vi "Thingworx_Read.vi"(8 "error in (no error)":errorcluster, 10 "Property In":T3, 11 "Device in":T2) -> (0 "error out":errorcluster, 2 "Property":T3, 3 "Device Out":T2)   [LabVIEW 2016]
uses:
  _subVIs/Device.ctl
  _subVIs/HTTPComm.ctl
panel:
  out "Comm":T1
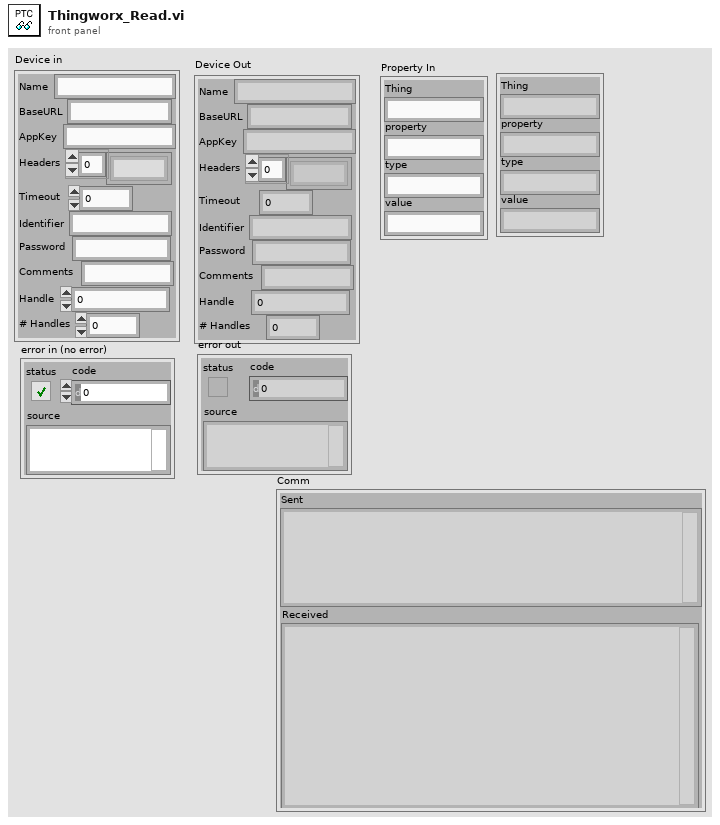
[diagram p1: front panel]
types:
  T1 = typedef "HTTPComm.ctl" = cluster{"url":string, "sent headers":string, "sent body":string, "headers":string, "body":string, "Sent":string, "Received":string}
  T2 = typedef "Device.ctl" = cluster{"Name":string, "BaseURL":string, "AppKey":string, "Headers":string[], "Timeout":i32, "Identifier":string, "Password":string, "Comments":string, "Handle":u32, "# Handles":i32}
  T3 = cluster{"Thing":string, "property":string, "type":string, "value":string}
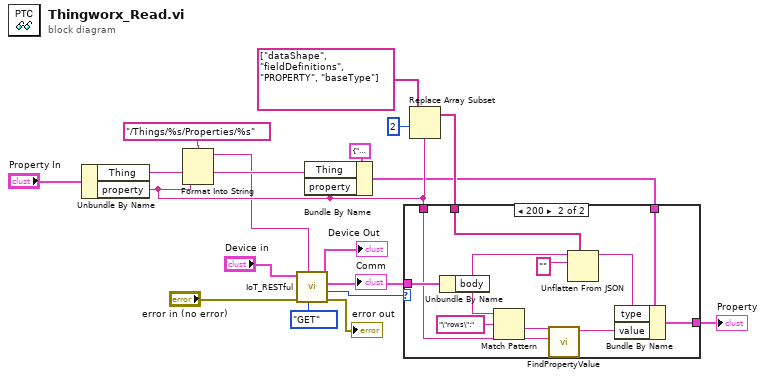
[diagram p0: block diagram]
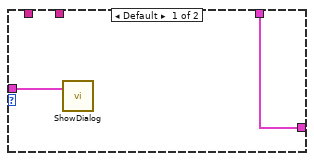
[diagram p2: hidden frame]
diagram:
  n1 = Unbundle By Name("Property In") -> ("Thing"=w11:string, "property"=w15:string)
  n2 = Format Into String(format string="/Things/%s/Properties/%s", w11, w15) -> (resulting string=w10:string)  [unwired: 2 in, 1 out]
  n3 = call "IoT_RESTful.vi"("Method"=enum16{"GET", "PUT", "POST", "MultiPOST"}."GET", "url"=w10, "error in"="error in (no error)", "Device In"="Device in") -> ("error out"=→"error out":errorcluster, "HTTP Code"=w17:i32, "Comm"=w7:T1, "Device Out"=→"Device Out":T2)  [unwired: 4 in]
  "Comm" <- w7
  n4 = Bundle By Name(cluster=T3 {"Thing"="", "property"="", "type"="", "value"=""} ("Property"), "Thing"=w11, "property"=w15) -> (w12:T3)
  n5 = Replace Array Subset(array=string[] ["dataShape", "fieldDefinitions", "PROPERTY", "baseType"] ("path"), new element=w15, index=2) -> (w16:string[])
  n6 = case shown="200" w17 {
    tunnel: w7 -> [w19 w31]
    tunnel: w12 -> [w20 w28]
    tunnel: [w20 w26] -> w2
    tunnel: w15 -> [_ w22]
    tunnel: w16 -> [_ w21]
    frame Default {
      n7 = call "ShowDialog.vi"("Comm"=w19) -> ()  [unwired: 11 in]
    }
    frame 200 {
      n8 = Unbundle By Name(w31) -> ("body"=w25:string)
      n9 = Match Pattern(string=w25, regular expression="\"rows\":") -> (after substring=w29:string)  [unwired: 1 in, 3 out]
      n10 = call "FindPropertyValue.vi"("property"=w22, "rows"=w29) -> ("value"=w27:string)  [unwired: 9 in]
      n11 = Unflatten From JSON(path=w21, JSON string=w25, type and defaults="" ("regular expression")) -> (value=w23:string)  [unwired: 4 in, 1 out]
      n12 = Bundle By Name(cluster=w28, "type"=w23, "value"=w27) -> (w26:T3)
    }
  }
  "Property" <- w2
